vi "Read Logic Datas.vi"(8 "error in (no error)":errorcluster, 10 "length":u32, 11 "buffer":string) -> (0 "error out":errorcluster, 2 "function return":u32, 3 "buffer out":string)   [LabVIEW 2021, in "vmmsolib.lvlib"]
doc: "DLL_API unsigned int WINAPI ReadLogicDatas(unsigned char* buffer, unsigned int length);"
uses:
  vmmsolib.lvlib
  vmmso.dll
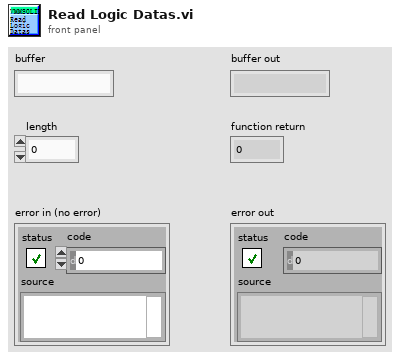
[diagram p1: front panel]
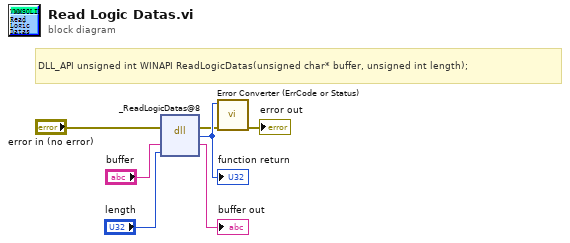
[diagram p0: block diagram]
diagram:
  # "DLL_API unsigned int WINAPI ReadLogicDatas(unsigned char* buffer, unsigned int length);"
  n1 = dll-call lib="D:/VmMsoSDK/demo-Labview/2021/vmmsolib/vmmso.*" fn="_ReadLogicDatas@8"(error in="error in (no error)", "buffer"="buffer", "length"="length") -> (error out=w2:errorcluster, w7:u32, "buffer"=→"buffer out":string)  [unwired: 3 in, 1 out]
  "function return" <- w7
  n2 = call "Error Converter (ErrCode or Status).vi"("error in (no error)"=w2, "error code"=w7) -> ("error out"=→"error out":errorcluster)  [unwired: 9 in]
